vi "Query Platform Format.vi"(8 "error in (no error)":errorcluster, 11 "VISA resource name":refnum<visa-resource-name>) -> (0 "error out":errorcluster, 1 "Length":i16, 2 "Type":string, 3 "VISA resource name out":refnum<visa-resource-name>)   [LabVIEW 2018, in "LTB-1.lvlib" / "3150.lvlib"]
doc: "Queries the format of the platform. The ASCII (Type) is returned when numeric data is transferred to ASCII bytes in interger, float or exponential representation, as appropriate."
uses:
  3150.lvlib
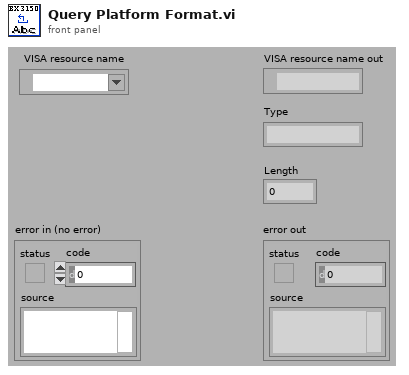
[diagram p1: front panel]
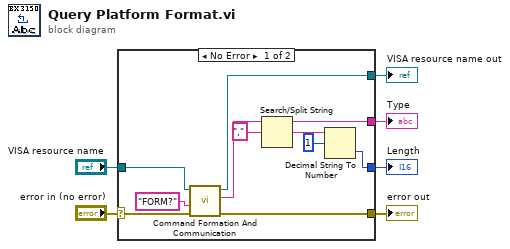
[diagram p0: block diagram]
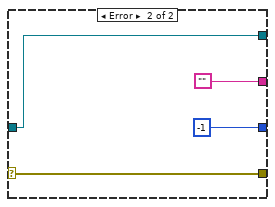
[diagram p2: hidden frame]
diagram:
  n1 = case shown="No Error" "error in (no error)" {
    selector: "error in (no error)" -> [w13 w21]
    tunnel: [w11 w20] -> w5
    tunnel: [w10 w21] -> w3
    tunnel: [w7 ""] -> w2
    tunnel: [w17 -1] -> w1
    tunnel: "VISA resource name" -> [w9 w20]
    frame No Error {
      n2 = call "Command Formation And Communication.vi"("error in (no error)"=w13, "Command"="FORM?", "VISA resource name"=w9) -> ("error out"=w10:errorcluster, "Response"=w12:string, "VISA resource name out"=w11:refnum<visa-resource-name>)  [unwired: 1 in, 5 out]
      n3 = Search/Split String(string=w12, search string/char (-)=",") -> (substring before match=w7:string, match + rest of string=w16:string)  [unwired: 2 out]
      n4 = Decimal String To Number(string=w16, offset=1 ("offset (0)")) -> (number=w17:i32)  [unwired: 2 out]
    }
    frame Error {
    }
  }
  "VISA resource name out" <- w5
  "error out" <- w3
  "Type" <- w2
  "Length" <- w1
